vi "Populate pressure constants array.vi"(1 "Occupied slot EEPROM values":T2[](array[typedef]), 2 "Active sensor indices":i32[](array[numeric])) -> (0 "Active pressure sensor constants":T1[](array[typedef]))   [LabVIEW 2015]
uses:
  Ctls/EEPROM page.ctl
  Ctls/Pressure sensor constants.ctl
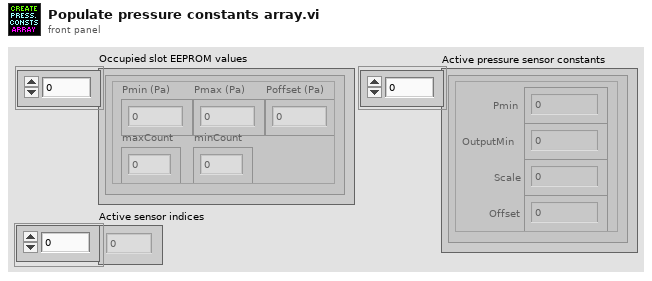
[diagram p1: front panel]
types:
  T1 = typedef "Pressure sensor constants.ctl" = cluster{"Pmin":sgl, "OutputMin":sgl, "Scale":sgl, "Offset":sgl}
  T2 = typedef "EEPROM page.ctl" = cluster{"Pmin (Pa)":sgl, "Pmax (Pa)":sgl, "maxCount":u16, "minCount":u16, "Poffset (Pa)":sgl}
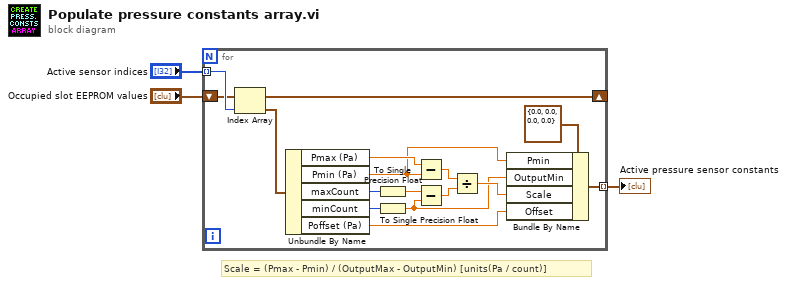
[diagram p0: block diagram]
diagram:
  # "Scale = (Pmax - Pmin) / (OutputMax - OutputMin) [units(Pa / count)]"
  n1 = for {
    tunnel: "Active sensor indices" -> [w18] mode=indexing
    shift-right: [w16] -> _
    shift-left: "Occupied slot EEPROM values" -> [w16]
    tunnel: [w12] -> w1 mode=indexing
    n2 = Index Array(array=w16, index=w18) -> (element=w15:T2)
    n3 = Unbundle By Name(w15) -> ("Pmax (Pa)"=w5:sgl, "Pmin (Pa)"=w4:sgl, "maxCount"=w8:u16, "minCount"=w14:u16, "Poffset (Pa)"=w13:sgl)
    n4 = To Single Precision Float(number=w8) -> (single precision float=w7:sgl)
    n5 = To Single Precision Float(number=w14) -> (single precision float=w6:sgl)
    n6 = Subtract(x=w5, y=w4) -> (x-y=w11:sgl)
    n7 = Subtract(x=w7, y=w6) -> (x-y=w10:sgl)
    n8 = Divide(x=w11, y=w10) -> (x/y=w9:sgl)
    n9 = Bundle By Name(cluster=T1 {"Pmin"=0.0, "OutputMin"=0.0, "Scale"=0.0, "Offset"=0.0} ("P constants"), "Pmin"=w4, "OutputMin"=w6, "Scale"=w9, "Offset"=w13) -> (w12:T1)
  }
  "Active pressure sensor constants" <- w1
